vi "Build_CommCluster_old.vi"(6 "reply body":string, 7 "Type":string="GET", 8 "reply headers":string, 9 "sent body":string, 10 "sent headers":string, 11 "url":string) -> (0 "Code":i32, 3 "Comm":T1)   [LabVIEW 2019]
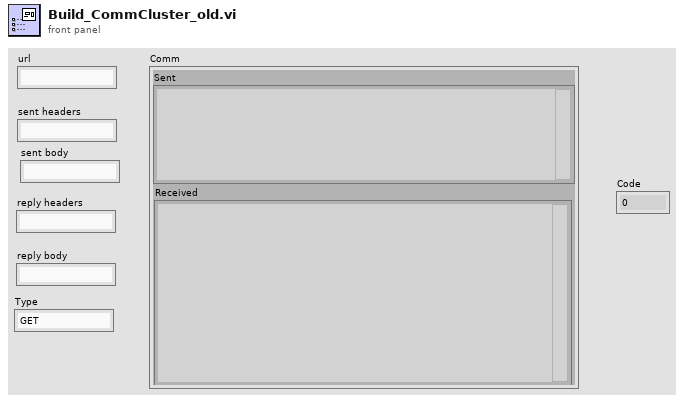
[diagram p1: front panel]
types:
  T1 = cluster{"url":string, "sent headers":string, "sent body":string, "headers":string, "body":string, "Sent":string, "Received":string}
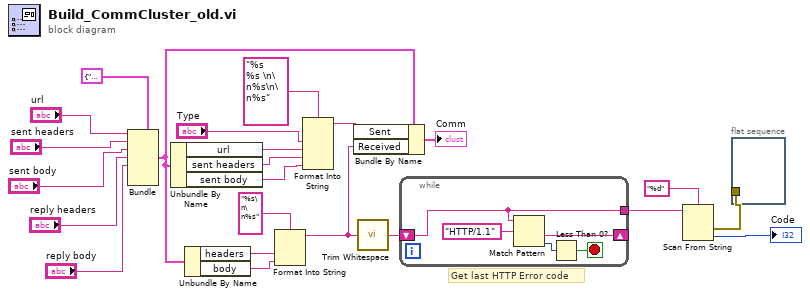
[diagram p0: block diagram]
diagram:
  # "Get last HTTP Error code"
  n1 = Bundle(cluster=T1 {"url"="", "sent headers"="", "sent body"="", "headers"="", "body"="", "Sent"="", "Received"=""} ("Comm"), "url"="url", "sent headers"="sent headers", "sent body"="sent body", "headers"="reply headers", "body"="reply body") -> (w21:T1)  [unwired: 2 in]
  n2 = Unbundle By Name(w21) -> ("url"=w17:string, "sent headers"=w18:string, "sent body"=w8:string)
  n3 = Unbundle By Name(w21) -> ("headers"=w19:string, "body"=w20:string)
  n4 = Format Into String(format string="%s\n\n%s", w19, w20) -> (resulting string=w3:string)  [unwired: 2 in, 1 out]
  n5 = Format Into String(format string="%s %s \n\n%s\n\n%s", "Type", w17, w18, w8) -> (resulting string=w22:string)  [unwired: 2 in, 1 out]
  n6 = Bundle By Name(cluster=w21, "Sent"=w22, "Received"=w3) -> (→"Comm":T1)
  n7 = call <vilib>:"Trim Whitespace.vi"("string"=w3) -> ("trimmed string"=w5:string)  [unwired: 1 in]
  n8 = while {
    shift-right: [w25] -> _
    shift-left: w5 -> [w24]
    tunnel: [w24] -> w6
    stop <- w27 stop-if-true
    n9 = Match Pattern(string=w24, regular expression="HTTP/1.1") -> (after substring=w25:string, offset past match=w26:i32)  [unwired: 1 in, 2 out]
    n10 = Less Than 0?(x=w26) -> (x < 0?=w27:bool)
  }
  n11 = Scan From String(format string="%d", input string=w6) -> (error out=w1:errorcluster, output 1=→"Code":i32)  [unwired: 3 in, 2 out]
  n12 = flat-sequence {
    tunnel: w1 -> [_]
    frame #0 {
    }
  }
